vi "registerReceivedMsgEvent.vi"(8 "error in (no error)":errorcluster, 11 "MonoCommunicator in":refnum<class "MonoCommunicator.lvclass">) -> (0 "error out":errorcluster, 2 "msgReceivedEvent":refnum<event-registration>, 3 "MonoCommunicator out":refnum<class "MonoCommunicator.lvclass">)   [LabVIEW 2016, in "MonoCommunicator.lvclass"]
uses:
  MonoCommunicator.lvclass
  MonoCommunicator.lvclass/MonoCommunicator.ctl
  ts_labview_tcp/TCPCommunicator/TCPCommunicator.lvclass/TCPCommunicator.ctl
  ts_labview_tcp/TCPComEvents/TCPComEvents.lvclass/TCPComEvents.ctl
  ts_labview_tcp/TCPServer/TCPServer.lvclass
  C:/Users/aanania/Documents/ts_monochromator_windows/ts_labview_tcp/TCPCommunicator/TCPCommunicator.lvclass
  ts_labview_tcp/TCPComEvents/TCPComEvents.lvclass
  ts_labview_tcp/TCPCommunicator/TCPCommunicator.lvclass
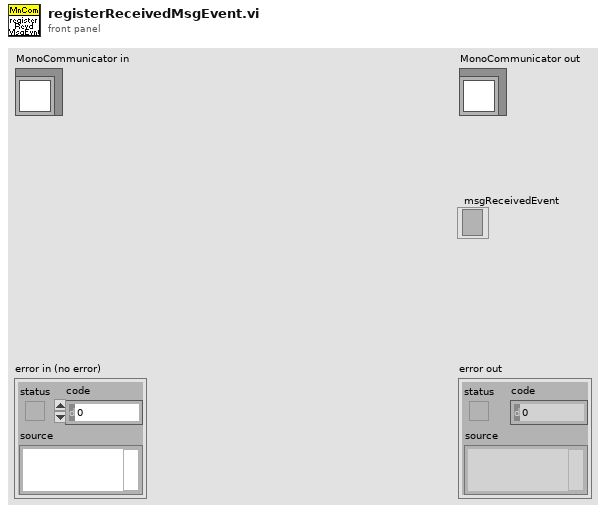
[diagram p1: front panel]
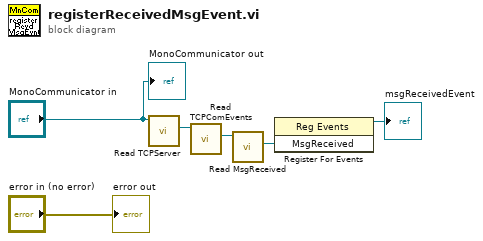
[diagram p0: block diagram]
diagram:
  n1 = call "Read TCPServer.vi"("MonoCommunicator in"="MonoCommunicator in") -> ("TCPServer.lvclass"=w4:refnum<class "TCPServer.lvclass">)  [unwired: 8 in, 2 out]
  n2 = call "Read TCPComEvents.vi"("TCPCommunicator in"=w4) -> ("TCPComEvents.lvclass"=w5:refnum<class "TCPComEvents.lvclass">)  [unwired: 8 in, 2 out]
  n3 = call "Read MsgReceived.vi"("TCPComEvents in"=w5) -> ("MsgReceived"=w2:refnum<user-event>)  [unwired: 8 in, 2 out]
  n4 = register-events(w2) -> (reference out=→"msgReceivedEvent":refnum<event-registration>)  [unwired: 2 in, 1 out]
  "error out" <- "error in (no error)"
  "MonoCommunicator out" <- "MonoCommunicator in"
